vi "CSGaussmeter.LimitFunction.vi"(0 "String":string, 5 "LIML":dbl, 7 "LIMU":dbl, 9 "Boolean":bool, 11 "error in":errorcluster) -> (6 "Answer":string, 15 "error out":errorcluster)   [LabVIEW 2014, in "CSGaussmeter.lvlib"]
uses:
  CSGaussmeter.lvlib
  instr.lib/FH_55/FH 55.lvlib
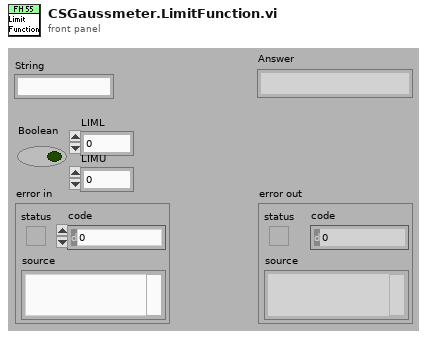
[diagram p1: front panel]
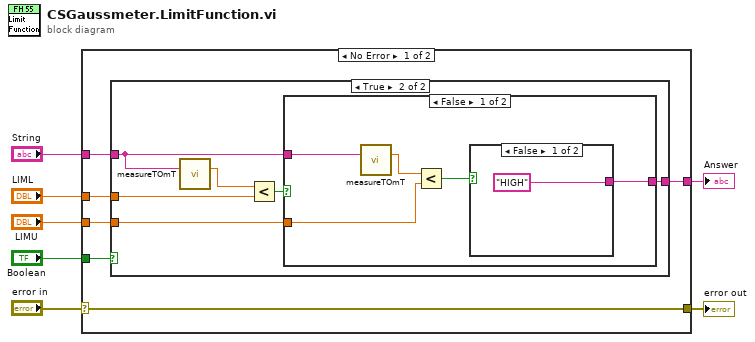
[diagram p0: block diagram]
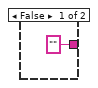
[diagram p2: hidden frame]
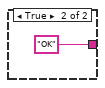
[diagram p3: hidden frame]
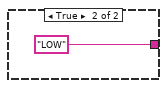
[diagram p4: hidden frame]
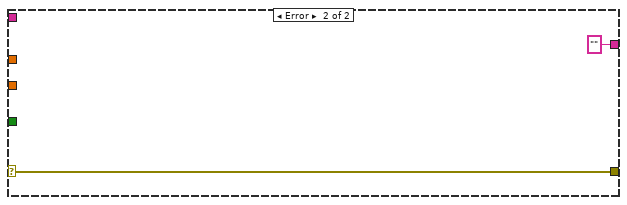
[diagram p5: hidden frame]
diagram:
  n1 = case shown="No Error" "error in" {
    selector: "error in" -> [w11 w29]
    tunnel: [w13 ""] -> w7
    tunnel: "String" -> [w12 _]
    tunnel: [w11 w29] -> w4
    tunnel: "Boolean" -> [w10 _]
    tunnel: "LIML" -> [w9 _]
    tunnel: "LIMU" -> [w8 _]
    frame No Error {
      n2 = case shown="True" w10 {
        tunnel: ["" w20] -> w13
        tunnel: w12 -> [_ w17]
        tunnel: w9 -> [_ w16]
        tunnel: w8 -> [_ w15]
        frame False {
        }
        frame True {
          n3 = call "measureTOmT.vi"("string"=w17) -> ("Numeric"=w18:dbl)  [unwired: 12 in, 2 out]
          n4 = Less?(x=w18, y=w16) -> (x < y?=w19:bool)
          n5 = case shown="False" w19 {
            tunnel: [w24 "LOW"] -> w20
            tunnel: w17 -> [w23 _]
            tunnel: w15 -> [w21 _]
            frame False {
              n6 = call "measureTOmT.vi"("string"=w23) -> ("Numeric"=w22:dbl)  [unwired: 12 in, 2 out]
              n7 = Less?(x=w22, y=w21) -> (x < y?=w25:bool)
              n8 = case shown="False" w25 {
                tunnel: ["HIGH" "OK"] -> w24
                frame False {
                }
                frame True {
                }
              }
            }
            frame True {
            }
          }
        }
      }
    }
    frame Error {
    }
  }
  "Answer" <- w7
  "error out" <- w4
